vi "Test-All-JoyStick.vi"() -> ()   [LabVIEW 2023]
doc: "This VI implements the framework and scheduler for your robotics program. It should not be necessary to modify the framework. You are expected to add your code to the VIs called from Robot Main - the ones located in the Team Code folder within the project."
uses:
  Robot Global Data.vi
  <vilib>/Rock Robotics/WPI/Simulation/Protocol/Devices/DriverStation/DS Update Ops.ctl
  <vilib>/Rock Robotics/WPI/DriverStation/WPI_DriverStationRobotMode2.ctl
  MNM/EminemStatesEnum.ctl
panel:
  out "Low Limit Switch":bool
  out "PosDeg":dbl format="%9.1f"
  out "Shoulder MotorOutDmd":dbl format="%9.2f"
  out "IntakeMtrOut":dbl
  in  "HaveNoteSensor":bool
  out "MNM State":T1=enum."13-AmpDone"
  out "MotorRPM Feed":dbl format="%#10.0f"
  out "MotorRPM Bot":dbl format="%#10.0f"
  out "MotorRPM Top":dbl format="%#10.0f"
  out "Robot Mode":T2
  in  "Finish":bool
  # "Sensor Simulation"
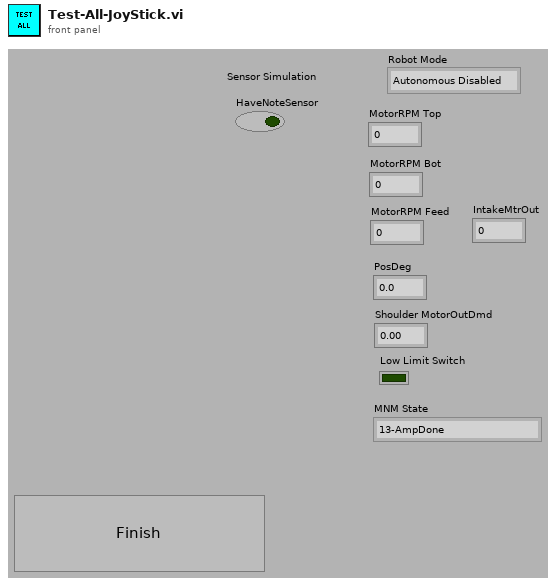
[diagram p1: front panel]
types:
  T1 = typedef "EminemStatesEnum.ctl" = enum16{"0-Init", "1-WaitForCmd", "2-Cancel", "3-ShootStart", "4-ShootRev", "5-RevUpStart", "6-ShootStartFeed&Timer", "7-ShootTimerOrSensorDone", "8-ShootDone", "9-AmpStart", "10-AmpUpToSpd?", "11-AmpStartFeed&Timer", "12-AmpTimerOrSensorDone", "13-AmpDone", "14-RevUpGetCmd"}
  T2 = typedef "WPI_DriverStationRobotMode2.ctl" = enum16{"Autonomous Disabled", "Autonomous Enabled", "Teleop Disabled", "Teleop Enabled", "Disconnected", "Finish", "Test Disabled", "Test Enabled", "Emergency Stopped"}
  T3 = typedef "WPI_DriverStationMatch Info.ctl" = cluster{"Autonomous Elapsed Seconds":dbl, "TeleOp Elapsed Seconds":dbl, "Disabled Elapsed Seconds":dbl, "Visited Autonomous":bool, "Visited TeleOp":bool, "Visited Disabled":bool, "Autonomous Settings":cluster{"Autonomous Style":enum16{"Iterative", "Independent"}, "VI Refnum":refnum<vi>}}
  T4 = typedef "WPI_DriverStationDerivedRobotMode.ctl" = enum16{"Init", "Execute", "Stop"}
  T5 = typedef "DS Update Ops.ctl" = enum16{"set enabled", "set autonomous", "set test", "set estop", "set fms", "set ds", "set control word", "set match_time", "set station", "set game data", "JSON update", "set name", "get", "transmit initial", "reset"}
  T6 = typedef "NetComm_ControlWord.ctl" = cluster{"Enabled":bool, "Autonomous":bool, "Test":bool, "E-Stop":bool, "FMS Attached":bool, "DS Attached":bool}
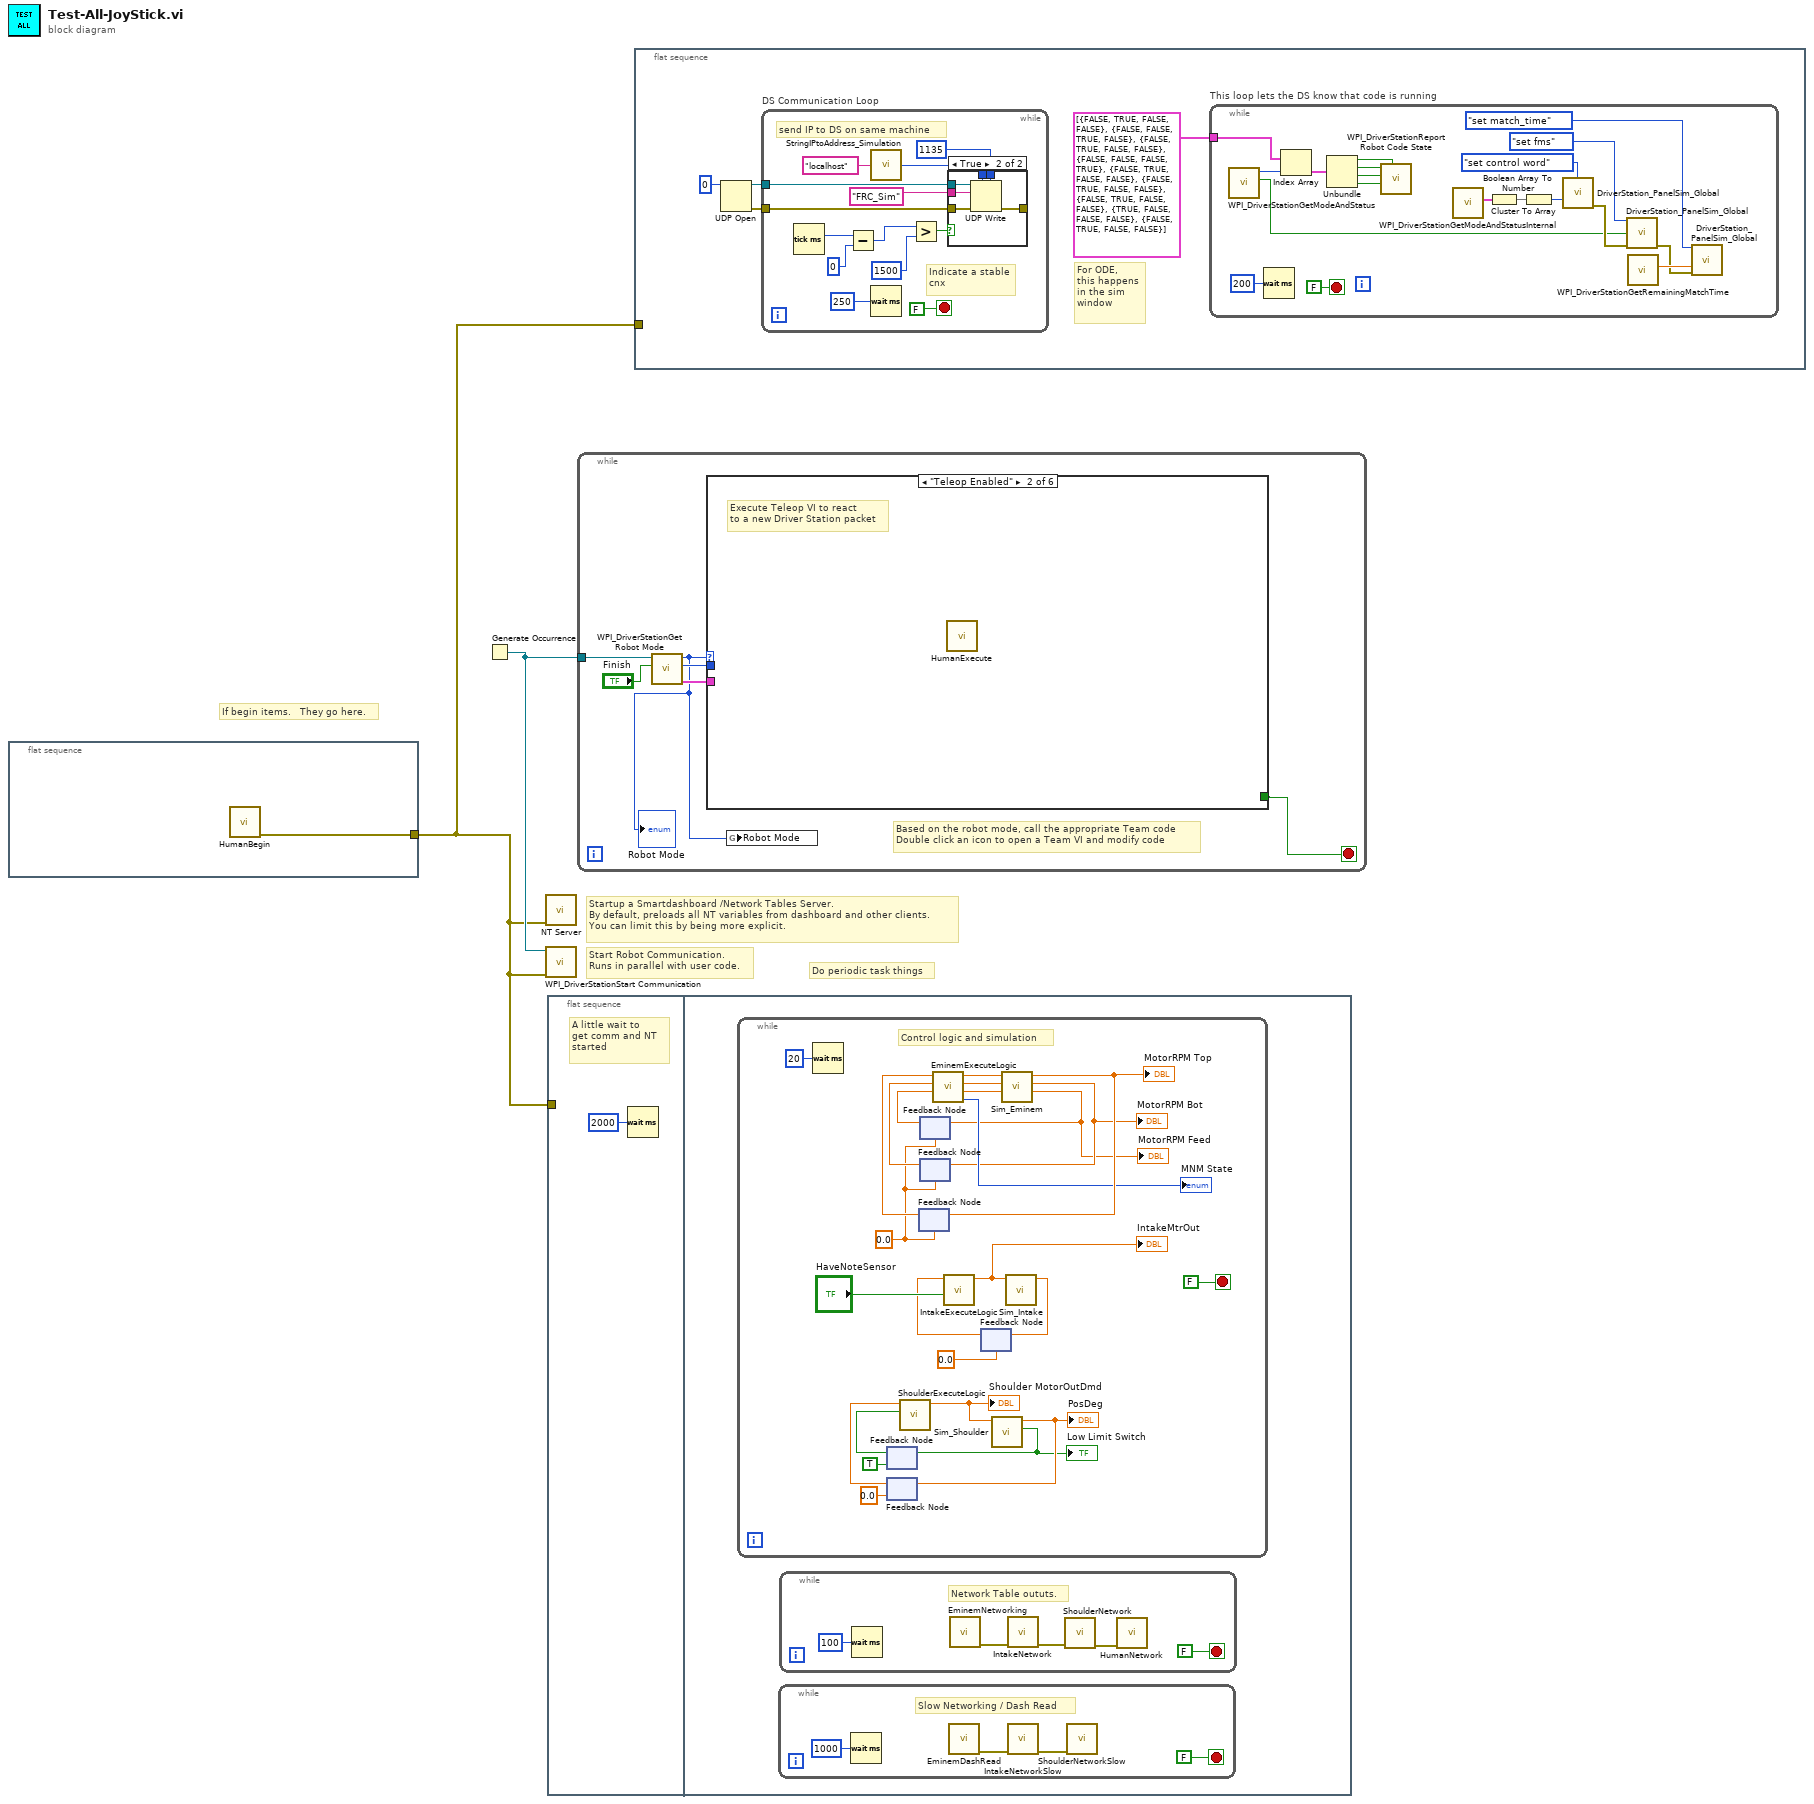
[diagram p0: block diagram]
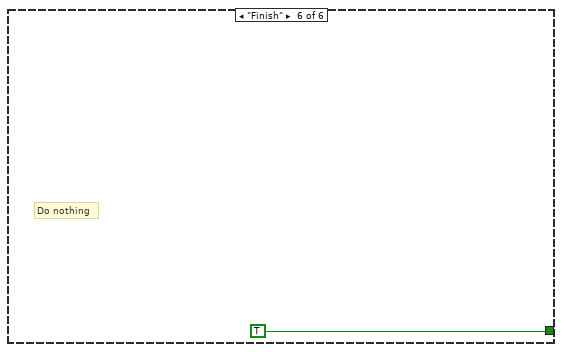
[diagram p6: hidden frame]
diagram:
  # "If begin items.   They go here."
  # "Do periodic task things"
  # "Startup a Smartdashboard /Network Tables Server.\nBy default, preloads all NT variables from dashboard and other clients.\nYou can limit this by being more explicit."
  # "Start Robot Communication.\nRuns in parallel with user code."
  n1 = flat-sequence {
    tunnel: [w3] -> w1
    frame #0 {
      n2 = call "HumanBegin.vi"() -> ("error out"=w3:errorcluster)  [unwired: 11 in]
    }
  }
  n3 = Generate Occurrence() -> (w2:refnum<k4>)
  n4 = call <vilib>:"NT Server.vi"("error in (no error)"=w1) -> ()  [unwired: 10 in, 1 out]
  n5 = call <vilib>:"WPI_DriverStationStart Communication.vi"("error in (no error)"=w1, "occurrence"=w2) -> ()  [unwired: 1 in, 9 out]
  n6 = flat-sequence {
    tunnel: w1 -> [_]
    frame #0 {
      # "A little wait to\nget comm and NT\nstarted"
      n7 = Wait (ms)(milliseconds to wait=u32 2000) -> ()  [unwired: 1 out]
    }
    frame #1 {
      n8 = while {
        stop <- FALSE stop-if-true
        w28 = 0.0 ("ArmPosDeg")
        # "Control logic and simulation"
        n9 = Wait (ms)(milliseconds to wait=u32 20) -> ()  [unwired: 1 out]
        n10 = feedback #1(TRUE ("Low Limit Switch")) -> (w16:bool)
        n11 = feedback #2(0.0 ("ArmPosDeg")) -> (w18:dbl)
        n12 = call "ShoulderExecuteLogic.vi"("LowLimitSwitch"=w16, "PositionDeg"=w18) -> ("MotorDemand"=w20:dbl)  [unwired: 8 in, 1 out]
        "Shoulder MotorOutDmd" <- w20
        n13 = feedback #3(w28) -> (w34:dbl)
        n14 = feedback #4(w28) -> (w27:dbl)
        n15 = feedback #5(w28) -> (w33:dbl)
        n16 = call "EminemExecuteLogic.vi"("Feed_Vel_RPM"=w27, "Shooter_Bottom_Vel_RPM"=w33, "Shooter_Top_Vel_RPM"=w34) -> ("Box states"=→"MNM State":T1, "Shooter_Feed_Motor_Out"=w31:dbl, "Shooter_Bottom_Motor_Out"=w32:dbl, "Shooter_Top_Motor_Out"=w36:dbl)  [unwired: 5 in]
        n17 = feedback #6(0.0 ("ArmPosDeg")) -> (w21:dbl)
        n18 = call "IntakeExecuteLogic.vi"("HaveNoteSensor"="HaveNoteSensor", "Sensor Velocity"=w21) -> ("MotorOutDmd"=w24:dbl)  [unwired: 9 in]
        "IntakeMtrOut" <- w24
        n19 = call "Sim_Shoulder.vi"("Motor Dmd"=w20) -> ("Low Limit Switch"=w17:bool, "ArmPosDeg"=w19:dbl)  [unwired: 8 in, 1 out]
        "PosDeg" <- w19
        "Low Limit Switch" <- w17
        n20 = feedback-in #1(w17) -> ()
        n21 = feedback-in #2(w19) -> ()
        n22 = call "Sim_Eminem.vi"("Motor Dmd C"=w31, "Motor Dmd B"=w32, "Motor Dmd A"=w36) -> ("MotorRPM C"=w26:dbl, "MotorRPM B"=w29:dbl, "MotorRPM A"=w35:dbl)  [unwired: 6 in]
        "MotorRPM Top" <- w35
        "MotorRPM Bot" <- w29
        "MotorRPM Feed" <- w26
        n23 = feedback-in #3(w35) -> ()
        n24 = feedback-in #4(w26) -> ()
        n25 = feedback-in #5(w29) -> ()
        n26 = call "Sim_Intake.vi"("Motor Dmd"=w24) -> ("MotorRPM"=w22:dbl)  [unwired: 10 in]
        n27 = feedback-in #6(w22) -> ()
      }
      n28 = while {
        stop <- FALSE stop-if-true
        # "Slow Networking / Dash Read"
        n29 = Wait (ms)(milliseconds to wait=u32 1000) -> ()  [unwired: 1 out]
        n30 = call "EminemDashRead.vi"() -> ("error out"=w6:errorcluster)  [unwired: 11 in]
        n31 = call "IntakeNetworkSlow.vi"("error in (no error)"=w6) -> ("error out"=w5:errorcluster)  [unwired: 10 in]
        n32 = call "ShoulderNetworkSlow.vi"("error in (no error)"=w5) -> ()  [unwired: 10 in, 1 out]
      }
      n33 = while {
        stop <- FALSE stop-if-true
        # "Network Table oututs."
        n34 = Wait (ms)(milliseconds to wait=u32 100) -> ()  [unwired: 1 out]
        n35 = call "EminemNetworking.vi"() -> ("error out"=w11:errorcluster)  [unwired: 11 in]
        n36 = call "IntakeNetwork.vi"("error in (no error)"=w11) -> ("error out"=w10:errorcluster)  [unwired: 10 in]
        n37 = call "ShoulderNetwork.vi"("error in (no error)"=w10) -> ("error out"=w9:errorcluster)  [unwired: 10 in]
        n38 = call "HumanNetwork.vi"("error in (no error)"=w9) -> ()  [unwired: 10 in, 1 out]
      }
    }
  }
  n39 = while {
    tunnel: w2 -> [w44]
    stop <- w39 stop-if-true
    # "Based on the robot mode, call the appropriate Team code\nDouble click an icon to open a Team VI and modify code"
    n40 = call <vilib>:"WPI_DriverStationGet Robot Mode.vi"("Finish"="Finish", "DS Occurrence"=w44) -> ("Match Info out"=w41:T3, "Call Context"=w43:T4, "Robot Mode"=w40:T2)  [unwired: 7 out]
    "Robot Mode" <- w40
    n41 = case shown="\"Teleop Enabled\"" w40 {
      tunnel: w43 -> [_ _ _ _ _ _]
      tunnel: w41 -> [_ _ _ _ _ _]
      tunnel: [_ _ _ _ _ TRUE] -> w39
      frame "Autonomous Enabled" {
        # "Do nothing...."
      }
      frame "Teleop Enabled" {
        # "Execute Teleop VI to react\nto a new Driver Station packet"
        n42 = call "HumanExecute.vi"() -> ()  [unwired: 11 in, 1 out]
      }
      frame "Test Disabled", "Test Enabled" {
        # "Do nothing"
      }
      frame "Autonomous Disabled", "Teleop Disabled" {
        # "Do nothing."
      }
      frame "Disconnected", Default {
        # "Driver Station packet didn't arrive.\nPossibly useful for diagnostics"
      }
      frame "Finish" {
        # "Do nothing"
      }
    }
    n43 = global write "Robot Global Data.vi" "Robot Mode"(w40) -> ()
  }
  n44 = flat-sequence {
    tunnel: w1 -> [_]
    frame #0 {
      # "For ODE,\nthis happens\nin the sim\nwindow"
      n45 = UDP Open(11:u16 0 ("port")) -> (port=w49:refnum<k16>, 0:w48:errorcluster)  [unwired: 4 in, 1 out]
      n46 = while "DS Communication Loop" {
        tunnel: w49 -> [w80]
        tunnel: w48 -> [w81]
        stop <- FALSE stop-if-true
        # "Indicate a stable\ncnx"
        # "send IP to DS on same machine"
        n47 = Tick Count (ms)() -> (millisecond timer value=w70:u32)
        n48 = Subtract(x=w70, y=u32 0) -> (x-y=w73:u32)
        n49 = call <vilib>:"StringIPtoAddress_Simulation.vi"("string IP"="localhost" ("DS IP 2")) -> ("address"=w77:u32)  [unwired: 14 in]
        n50 = Wait (ms)(milliseconds to wait=u32 250) -> ()  [unwired: 1 out]
        n51 = Greater?(x=w73, y=u32 1500 ("milliseconds to wait")) -> (0:w71:bool)
        n52 = case shown="True" w71 {
          tunnel: w81 -> [_ w87]
          tunnel: w80 -> [_ w86]
          tunnel: "FRC_Sim" ("data in") -> [_ w85]
          tunnel: w77 -> [_ w84]
          tunnel: [_ w83] -> _
          tunnel: u16 1135 ("port") -> [_ w82]
          frame False {
          }
          frame True {
            n53 = UDP Write(address=w84, port or service name=w82, connection ID=w86, data in=w85, 8:w87) -> (error out=w83:errorcluster)  [unwired: 1 in, 1 out]
          }
        }
      }
      n54 = while "This loop lets the DS know that code is running" {
        tunnel: cluster{bool, bool, bool, bool}[] [{FALSE, TRUE, FALSE, FALSE}, {FALSE, FALSE, TRUE, FALSE}, {FALSE, TRUE, FALSE, FALSE}, {FALSE, FALSE, FALSE, TRUE}, {FALSE, TRUE, FALSE, FALSE}, {FALSE, TRUE, FALSE, FALSE}, {FALSE, TRUE, FALSE, FALSE}, {TRUE, FALSE, FALSE, FALSE}, {FALSE, TRUE, FALSE, FALSE}] -> [w67]
        stop <- FALSE stop-if-true
        n55 = call <vilib>:"WPI_DriverStationGetModeAndStatus.vi"() -> ("FMS Attached"=w50:bool, "Robot Mode"=w61:T2)  [unwired: 10 in]
        n56 = Wait (ms)(milliseconds to wait=u32 200) -> ()  [unwired: 1 out]
        n57 = Index Array(array=w67, index=w61) -> (element=w62:cluster{bool, bool, bool, bool})
        n58 = Unbundle(w62) -> (w68:bool, w60:bool, w65:bool, w64:bool)
        n59 = call <vilib>:"WPI_DriverStationReport Robot Code State.vi"("Test"=w68, "TeleOp"=w64, "Autonomous"=w65, "Disabled"=w60) -> ()  [unwired: 7 in, 1 out]
        n60 = call <vilib>:"WPI_DriverStationGetModeAndStatusInternal.vi"() -> ("Control Word"=w58:T6)  [unwired: 10 in, 1 out]
        n61 = Cluster To Array(cluster=w58) -> (array=w57:bool[])
        n62 = Boolean Array To Number(Boolean array=w57) -> (number=w56:u32)
        n63 = call <vilib>:"DriverStation_PanelSim_Global.vi"("menu"=DS_Update_Ops."set control word", "Numeric Value"=w56) -> ("error out"=w54:errorcluster)  [unwired: 12 in, 1 out]
        n64 = call <vilib>:"DriverStation_PanelSim_Global.vi"("menu"=DS_Update_Ops."set fms", "Value Set"=w50, "error in (no error)"=w54) -> ("error out"=w51:errorcluster)  [unwired: 11 in, 1 out]
        n65 = call <vilib>:"WPI_DriverStationGetRemainingMatchTime.vi"() -> ("Match Time(s)"=w52:sgl)  [unwired: 10 in, 1 out]
        n66 = call <vilib>:"DriverStation_PanelSim_Global.vi"("menu"=DS_Update_Ops."set match_time", "Numeric Value"=w52, "error in (no error)"=w51) -> ()  [unwired: 11 in, 2 out]
      }
    }
  }
